vi "read(sub).vi"(3 "errorin":errorcluster, 4 "writestring":string="R0003", 5 "readdelay":u32=500, 6 "resourcein":refnum<visa-resource-name>) -> (0 "errorout":errorcluster, 1 "readstring":string, 2 "resourceout":refnum<visa-resource-name>)   [LabVIEW 2015]
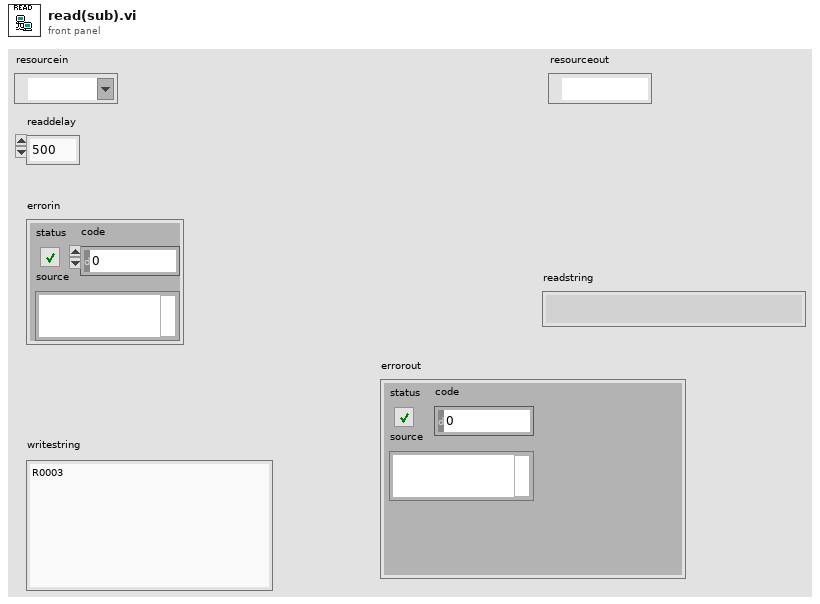
[diagram p1: front panel]
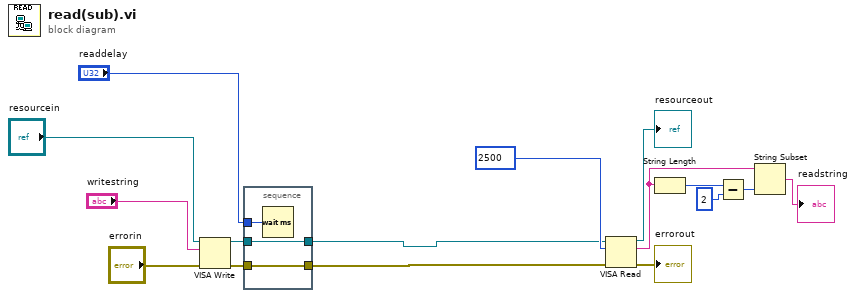
[diagram p0: block diagram]
diagram:
  n1 = VISA Write(VISA resource name="resourcein", write buffer="writestring", error in (no error)="errorin") -> (VISA resource name out=w5:refnum<visa-resource-name>, error out=w4:errorcluster)  [unwired: 1 out]
  n2 = stacked-sequence {
    tunnel: w4 -> [w19]
    tunnel: [w19] -> w1
    tunnel: w5 -> [w18]
    tunnel: [w18] -> w2
    tunnel: "readdelay" -> [w17]
    frame #0 {
      n3 = Wait (ms)(milliseconds to wait=w17) -> ()  [unwired: 1 out]
    }
  }
  n4 = VISA Read(VISA resource name=w2, byte count=u32 2500, error in (no error)=w1) -> (VISA resource name out=→"resourceout":refnum<visa-resource-name>, read buffer=w16:string, error out=→"errorout":errorcluster)  [unwired: 1 out]
  n5 = String Length(string=w16) -> (length=w14:i32)
  n6 = Subtract(x=w14, y=2 ("x")) -> (x-y=w15:i32)
  n7 = String Subset(string=w16, length (rest)=w15) -> (substring=→"readstring":string)  [unwired: 1 in]
